vi "writeEOD.vi"(8 "file path (use dialog)":path, 11 "Cluster":T1) -> (0 "error out":errorcluster, 3 "Iteration Count":i32)   [LabVIEW 2014]
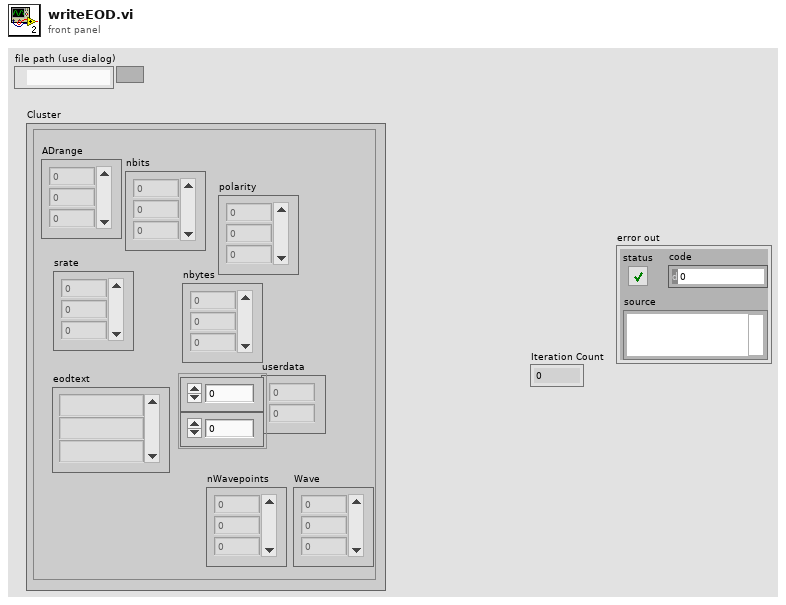
[diagram p1: front panel]
types:
  T1 = cluster{"eodtext":string[], "nbits":i8[], "nbytes":i8[], "polarity":i8[], "userdata":dbl[][], "ADrange":dbl[], "srate":u32[], "nWavepoints":u32[], "Wave":i16[]}
  T2 = enum16{"big-endian, network order", "native, host order", "little-endian"}
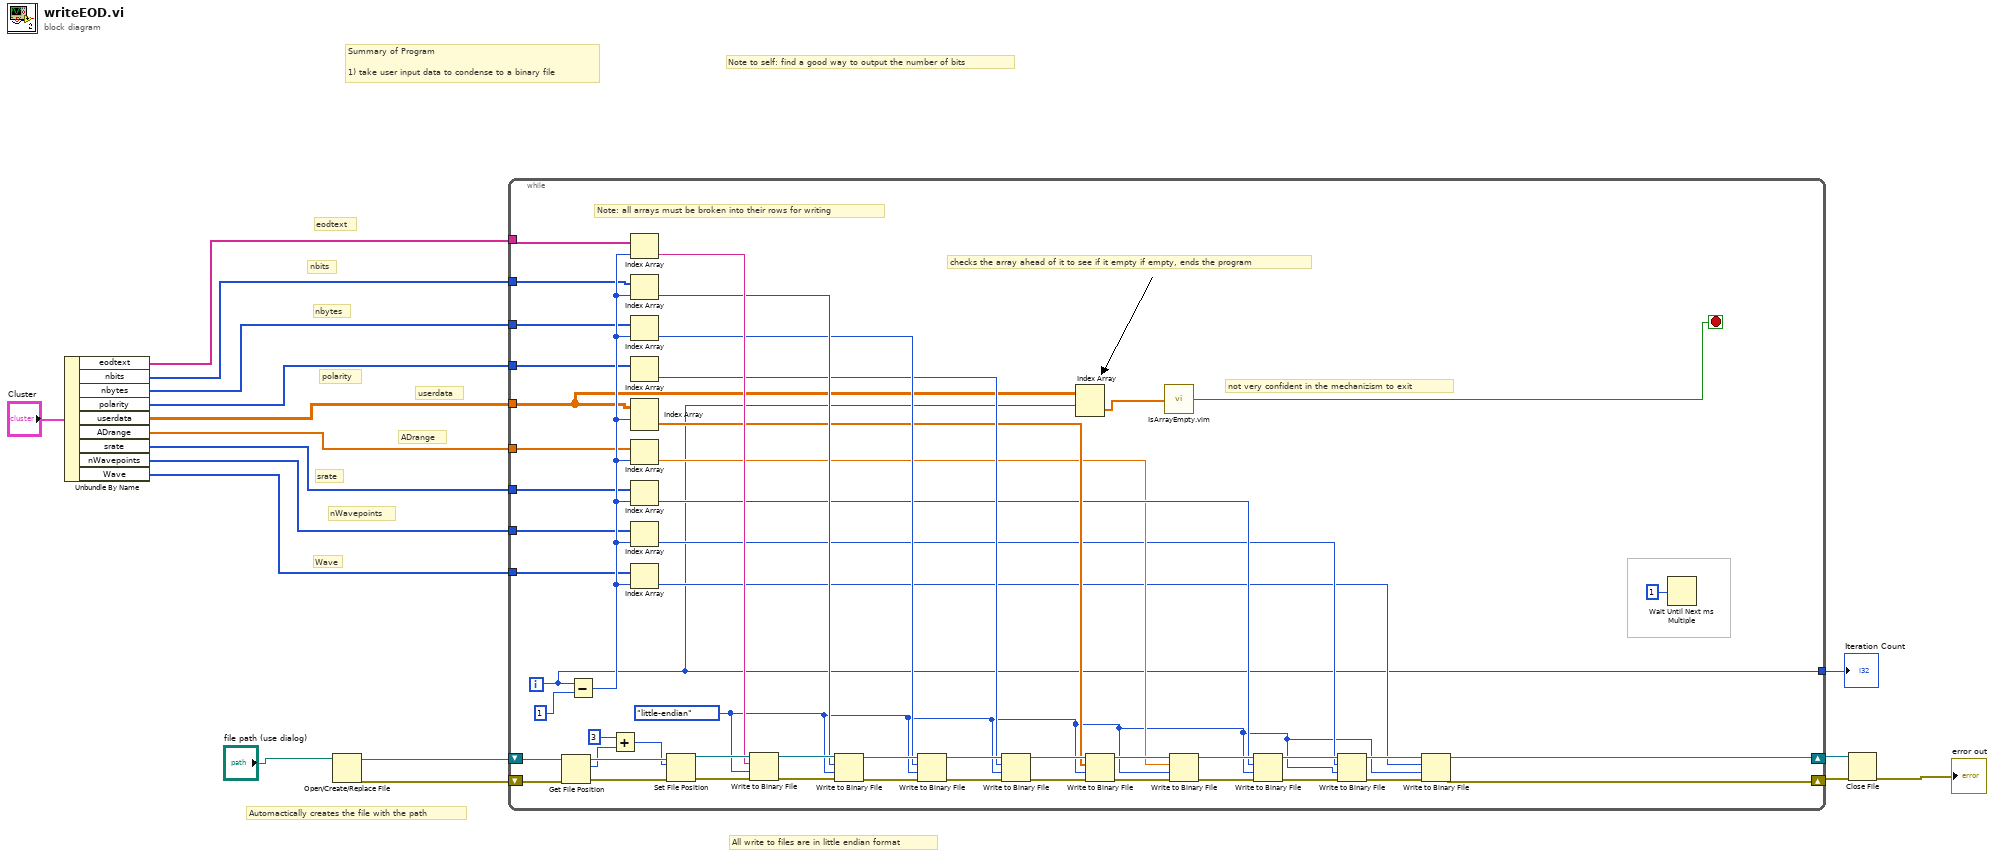
[diagram p0: block diagram]
diagram:
  # "All write to files are in little endian format"
  # "Wave"
  # "nWavepoints"
  # "ADrange"
  # "srate"
  # "userdata"
  # "polarity"
  # "nbytes"
  # "nbits"
  # "eodtext"
  # "Automactically creates the file with the path"
  # "Note to self: find a good way to output the number of bits"
  # "Summary of Program\n\n1) take user input data to condense to a binary file"
  n1 = Unbundle By Name("Cluster") -> ("eodtext"=w9:string[], "nbits"=w8:i8[], "nbytes"=w7:i8[], "polarity"=w6:i8[], "userdata"=w5:dbl[][], "ADrange"=w4:dbl[], "srate"=w3:u32[], "nWavepoints"=w2:u32[], "Wave"=w1:i16[])
  n2 = Open/Create/Replace File(file path (use dialog)="file path (use dialog)") -> (refnum out=w16:refnum<file>, error out=w15:errorcluster)  [unwired: 5 in, 1 out]
  n3 = while {
    shift-right: [w33] -> w14
    shift-left: w16 -> [w69]
    shift-right: [w32] -> w13
    shift-left: w15 -> [w68]
    tunnel: [w29] -> w12
    tunnel: w9 -> [w27]
    tunnel: w8 -> [w26]
    tunnel: w7 -> [w25]
    tunnel: w6 -> [w24]
    tunnel: w5 -> [w19]
    tunnel: w4 -> [w23]
    tunnel: w3 -> [w22]
    tunnel: w2 -> [w21]
    tunnel: w1 -> [w20]
    i -> [w29]
    stop <- w28 stop-if-true
    w31 = T2."little-endian" ("byte order (0:big-endian, network order)")
    # "not very confident in the mechanizism to exit"
    # "checks the array ahead of it to see if it empty if empty, ends the program"
    # "Note: all arrays must be broken into their rows for writing"
    n4 = Get File Position(4:w68, 7:w69) -> (0:w66:errorcluster, 2:w65:i64, 3:w67:refnum<file>)
    n5 = Subtract(x=w29, y=1) -> (x-y=w42:i32)
    n6 = Add(x=i64 3, y=w65) -> (x+y=w63:i64)
    n7 = Index Array(array=w27, index=w42) -> (element=w59:string)
    n8 = Index Array(array=w26, index=w42) -> (element=w41:i8)
    n9 = Index Array(array=w25, index=w42) -> (element=w40:i8)
    n10 = Index Array(array=w24) -> (element=w39:i8)  [unwired: 1 in]
    n11 = Index Array(array=w19, index (row)=w42) -> (element=w38:dbl[])  [unwired: 1 in]
    n12 = Index Array(array=w23, index=w42) -> (element=w36:dbl)
    n13 = Index Array(array=w22, index=w42) -> (element=w37:u32)
    n14 = Index Array(array=w21, index=w42) -> (element=w35:u32)
    n15 = Index Array(array=w20, index=w42) -> (element=w34:i16)
    n16 = Set File Position(offset (in bytes) (0)=w63, refnum=w67, error in=w66) -> (refnum out=w62:refnum<file>, error out=w61:errorcluster)  [unwired: 1 in]
    n17 = Write to Binary File(file (use dialog)=w62, data=w59, error in=w61, 9:w31) -> (refnum out=w58:refnum<file>, error out=w57:errorcluster)  [unwired: 2 in, 1 out]
    n18 = Write to Binary File(file (use dialog)=w58, data=w41, error in=w57, 9:w31) -> (refnum out=w55:refnum<file>, error out=w56:errorcluster)  [unwired: 2 in, 1 out]
    n19 = Write to Binary File(file (use dialog)=w55, data=w40, error in=w56, 9:w31) -> (refnum out=w54:refnum<file>, error out=w53:errorcluster)  [unwired: 2 in, 1 out]
    n20 = Write to Binary File(file (use dialog)=w54, data=w39, error in=w53, 9:w31) -> (refnum out=w51:refnum<file>, error out=w52:errorcluster)  [unwired: 2 in, 1 out]
    n21 = Index Array(array=w19, index (row)=w29) -> (element=w18:dbl[])  [unwired: 1 in]
    n22 = Write to Binary File(file (use dialog)=w51, data=w38, error in=w52, 9:w31) -> (refnum out=w50:refnum<file>, error out=w49:errorcluster)  [unwired: 2 in, 1 out]
    n23 = call <userlib>:"IsArrayEmpty.vim"("Array"=w18) -> ("empty"=w28:bool)
    n24 = Write to Binary File(file (use dialog)=w50, data=w36, error in=w49, 9:w31) -> (refnum out=w48:refnum<file>, error out=w47:errorcluster)  [unwired: 2 in, 1 out]
    n25 = Write to Binary File(file (use dialog)=w48, data=w37, error in=w47, 9:w31) -> (refnum out=w46:refnum<file>, error out=w45:errorcluster)  [unwired: 2 in, 1 out]
    n26 = Write to Binary File(file (use dialog)=w46, data=w35, error in=w45, 9:w31) -> (refnum out=w44:refnum<file>, error out=w43:errorcluster)  [unwired: 2 in, 1 out]
    n27 = Write to Binary File(file (use dialog)=w44, data=w34, error in=w43, 9:w31) -> (refnum out=w33:refnum<file>, error out=w32:errorcluster)  [unwired: 2 in, 1 out]
    n28 = Wait Until Next ms Multiple(millisecond multiple=u32 1) -> ()  [unwired: 1 out]
  }
  "Iteration Count" <- w12
  n29 = Close File(refnum=w14, error in=w13) -> (error out=→"error out":errorcluster)  [unwired: 1 out]
